vi "Configure Power Measurement List Parameter Set.vi"(7 "Parameter Set":dbl[](array[numeric]), 8 "error in (no error)":errorcluster, 9 "List Length (10)":i32=10, 10 "Instance (1)":i32=1, 11 "VISA resource name":refnum<visa-resource-name>) -> (0 "error out":errorcluster, 3 "VISA resource name out":refnum<visa-resource-name>)   [LabVIEW 2020, in "Rohde&Schwarz CMXP GPRF.lvlib"]
doc: "Selects the parameter set for all frequency/level step.\n\nAttribute:\nRSCMXPGPRF_ATTR_POWER_MEASUREMENT_LIST_PARAMETER_SET\n\nRemote-control command:\nCONFigure:GPRF:MEAS<i>:POWer:LIST:PSET:ALL"
uses:
  <instrlib>/Rohde&Schwarz CMXP GPRF/Rohde&Schwarz CMXP GPRF.lvlib
  <instrlib>/Rohde&Schwarz CMXP GPRF/Private/rsidr_core.llb/rsidr_core.lvlib
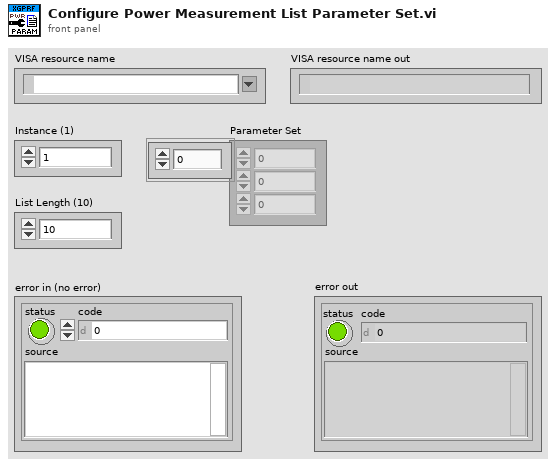
[diagram p1: front panel]
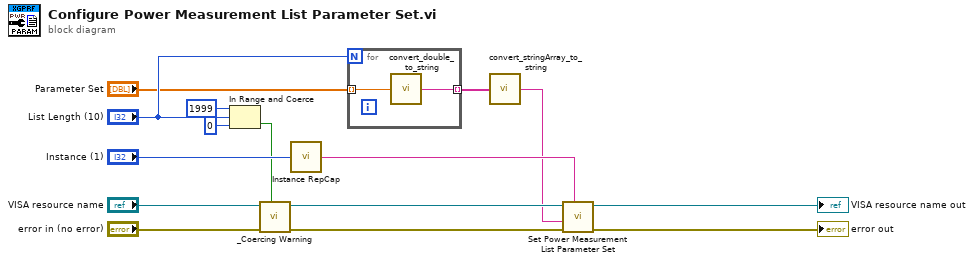
[diagram p0: block diagram]
diagram:
  n1 = In Range and Coerce(upper limit=1999, x="List Length (10)", lower limit=0) -> (In Range?=w2:bool)  [unwired: 1 out]
  n2 = call <instrlib>:"_Coercing Warning.vi"("In Range?"=w2, "error in (no error)"="error in (no error)", "VISA resource name"="VISA resource name") -> ("error out"=w8:errorcluster, "VISA resource name out"=w7:refnum<visa-resource-name>)  [unwired: 7 in]
  n3 = call <instrlib>:"Instance RepCap.vi"("Instance in"="Instance (1)") -> ("Instance out"=w4:string)
  n4 = for {
    N: "List Length (10)" -> [_]
    tunnel: "Parameter Set" -> [w17] mode=indexing
    tunnel: [w16] -> w9 mode=indexing
    n5 = call <instrlib>:"convert_double_to_string.vi"("double in"=w17) -> ("string out"=w16:string)  [unwired: 4 in]
  }
  n6 = call <instrlib>:"convert_stringArray_to_string.vi"("string array in"=w9) -> ("string out"=w1:string)  [unwired: 4 in]
  n7 = call "Set Power Measurement List Parameter Set"("Repeated Capabilities"=w4, "error in (no error)"=w8, "Power Measurement List Parameter Set ()"=w1, "instrument handle"=w7) -> ("error out"=→"error out":errorcluster, "instrument handle out"=→"VISA resource name out":refnum<visa-resource-name>)  [unwired: 6 in]
